vi "Resolve File Conflicts.vi"(8 "error in (no error)":errorcluster, 10 "Instance File Path in":path, 11 "Log File Specification in":refnum<class "Log File Specification.lvclass">) -> (0 "error out":errorcluster, 1 "Operation":T1, 2 "Instance File Path out":path, 3 "Log File Specification out":refnum<class "Log File Specification.lvclass">)   [LabVIEW 2012, in "Waveform Data Logger Shared.lvlib" / "Log File Specification.lvclass"]
doc: "This VI resolves the conflict if the specified file already exists according to the given File Conflict Operation. If Create Unique File Path is specified and the file already exists, the file path has an incrementing number appended to it until a new file path is found. The Filename Offset value is used as the first try for this incrementing value."
uses:
  Log File Specification.lvclass
  Engine/Classes/Logs/Log Files/Log File/Operation.ctl
  Log File Specification.lvclass/Log File Specification.ctl
  Engine/Classes/Logs/Log Files/Log File/Log File.lvclass
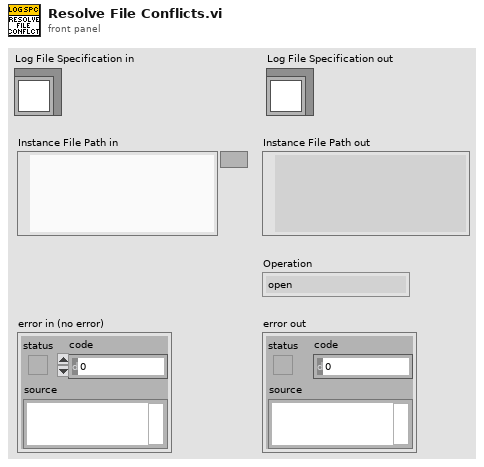
[diagram p1: front panel]
types:
  T1 = typedef "Waveform Data Logger Engine.lvlib/Log File.lvclass/Operation.ctl" = enum16{"open", "open or create", "create or replace", "create", "open (read-only)"}
  T2 = typedef "Waveform Data Logger Shared.lvlib/Log File Specification.lvclass/File Conflict Operation.ctl" = enum16{"Create Unique File Path", "Append to Existing", "Overwrite Existing"}
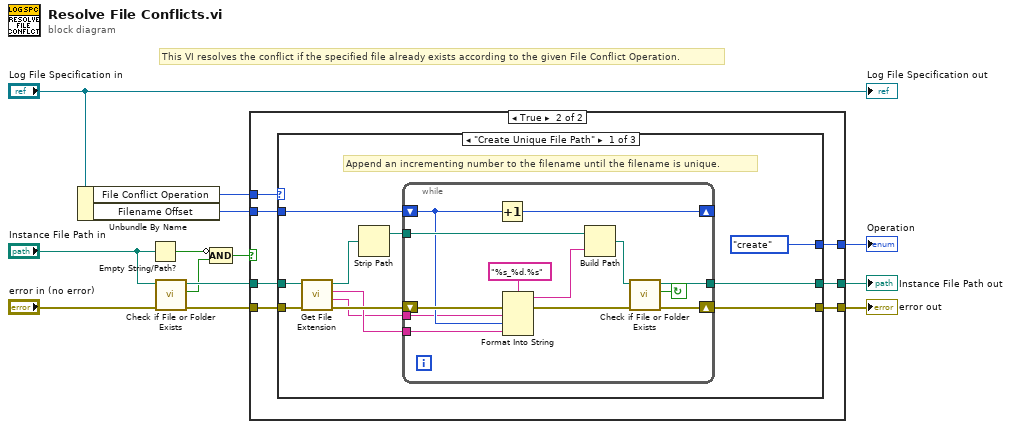
[diagram p0: block diagram]
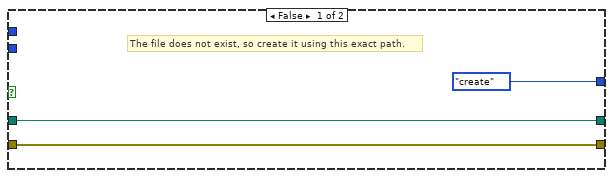
[diagram p2: hidden frame]
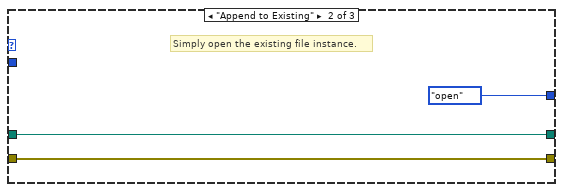
[diagram p3: hidden frame]
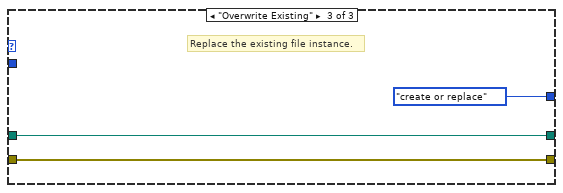
[diagram p4: hidden frame]
diagram:
  # "This VI resolves the conflict if the specified file already exists according to the given File Conflict Operation."
  n1 = Unbundle By Name("Log File Specification in") -> ("File Conflict Operation"=w2:T2, "Filename Offset"=w1:i32)
  n2 = Empty String/Path?(string/path="Instance File Path in") -> (empty?=w10:bool)
  n3 = call <vilib>:"Check if File or Folder Exists.vi"("error in (no error)"="error in (no error)", "path"="Instance File Path in") -> ("error out"=w8:errorcluster, "file or folder exists?"=w4:bool, "dup path"=w7:path)  [unwired: 7 in]
  n4 = Compound Arithmetic op=AND(invert w10, w4) -> (w11:bool)
  n5 = case shown="True" w11 {
    tunnel: w7 -> [w16 w21]
    tunnel: w8 -> [w15 w22]
    tunnel: [w16 w20] -> w12
    tunnel: [w15 w19] -> w5
    tunnel: w2 -> [_ w23]
    tunnel: [Operation."create" ("Operation") w18] -> w13
    tunnel: w1 -> [_ w17]
    frame False {
      # "The file does not exist, so create it using this exact path."
    }
    frame True {
      n6 = case shown="\"Create Unique File Path\"" w23 {
        tunnel: w22 -> [w32 w49 w52]
        tunnel: w21 -> [w33 w50 w53]
        tunnel: [w27 w50 w53] -> w20
        tunnel: [w26 w49 w52] -> w19
        tunnel: [Operation."create" ("Operation") Operation."open" ("Operation") Operation."create or replace" ("Operation")] -> w18
        tunnel: w17 -> [w25 _ _]
        frame "Create Unique File Path" {
          # "Append an incrementing number to the filename until the filename is unique."
          n7 = call <vilib>:"Get File Extension.vi"("error in (no error)"=w32, "file"=w33) -> ("error out"=w34:errorcluster, "filename without extension"=w24:string, "lowercase file extension"=w29:string, "dup file"=w31:path)  [unwired: 6 in]
          n8 = Strip Path(path=w31) -> (stripped path=w28:path)  [unwired: 1 out]
          n9 = while {
            tunnel: w29 -> [w44]
            tunnel: w24 -> [w35]
            tunnel: w28 -> [w42]
            tunnel: [w38] -> w27
            shift-right: [w37] -> w26
            shift-left: w34 -> [w46]
            shift-right: [w47] -> _
            shift-left: w25 -> [w36]
            stop <- w39 continue-if-true
            n10 = Increment(x=w36) -> (x+1=w47:i32)
            n11 = Format Into String(format string="%s_%d.%s", error in=w46, w35, w36, w44) -> (resulting string=w41:string, error out=w43:errorcluster)  [unwired: 1 in]
            n12 = Build Path(base path=w42, name or relative path=w41) -> (appended path=w40:path)
            n13 = call <vilib>:"Check if File or Folder Exists.vi"("error in (no error)"=w43, "path"=w40) -> ("error out"=w37:errorcluster, "file or folder exists?"=w39:bool, "dup path"=w38:path)  [unwired: 7 in]
          }
        }
        frame "Append to Existing" {
          # "Simply open the existing file instance."
        }
        frame "Overwrite Existing" {
          # "Replace the existing file instance."
        }
      }
    }
  }
  "Operation" <- w13
  "Instance File Path out" <- w12
  "error out" <- w5
  "Log File Specification out" <- "Log File Specification in"
